vi "Create XY Graph from Concatenated Waveform.vi"(0 "waveform t0 array":dbl[](array[numeric]), 5 "waveform dt array":dbl[](array[numeric]), 7 "waveform length array":i32[](array[numeric]), 9 "concatenated waveform Y":dbl[](array[numeric])) -> (4 "XY Graph Array":cluster{"time":dbl[], "waveform":dbl[]}[](array[cluster]))   [LabVIEW 2021, in "PMIC Common.lvlib"]
uses:
  PMIC Common.lvlib
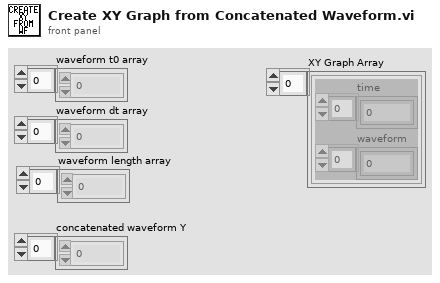
[diagram p1: front panel]
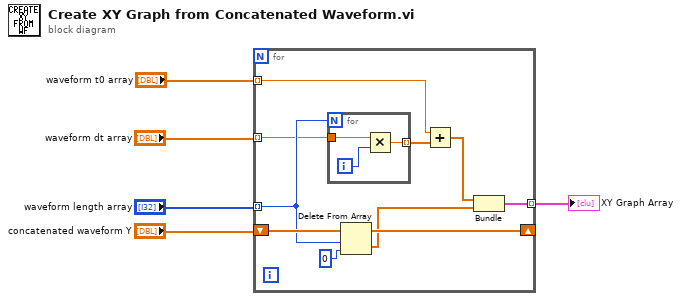
[diagram p0: block diagram]
diagram:
  n1 = for {
    tunnel: "waveform t0 array" -> [w6] mode=indexing
    tunnel: "waveform dt array" -> [w11] mode=indexing
    shift-right: [w14] -> _
    shift-left: "concatenated waveform Y" -> [w15]
    tunnel: "waveform length array" -> [w12] mode=indexing
    tunnel: [w7] -> w1 mode=indexing
    n2 = for {
      N: w12 -> [_]
      tunnel: w11 -> [w17]
      tunnel: [w16] -> w10 mode=indexing
      i -> [w18]
      n3 = Multiply(x=w17, y=w18) -> (x*y=w16:dbl)
    }
    n4 = Delete From Array(array=w15, length=w12, index=0) -> (deleted portion=w8:dbl[], array with subset deleted=w14:dbl[])
    n5 = Add(x=w6, y=w10) -> (x+y=w9:dbl[])
    n6 = Bundle(w9, "concatenated waveform Y"=w8) -> (w7:cluster{dbl[], "concatenated waveform Y":dbl[]})  [unwired: 1 in]
  }
  "XY Graph Array" <- w1
